vi "compute_statistics_data.vi"() -> ()   [LabVIEW 2020]
uses:
  StatisticsData.ctl
  ComputePhaseSet.lvclass
  WavefrontReconstructionMode.ctl
  HasoData.lvclass
  Phase.lvclass
  Pupil.lvclass
panel:
  out "Wavefront":sgl[][](graph)
  in  "Haso slopes file name":string="Data\\data_phase_computation.has"
  out "error out":errorcluster
  out "Statistics":T1
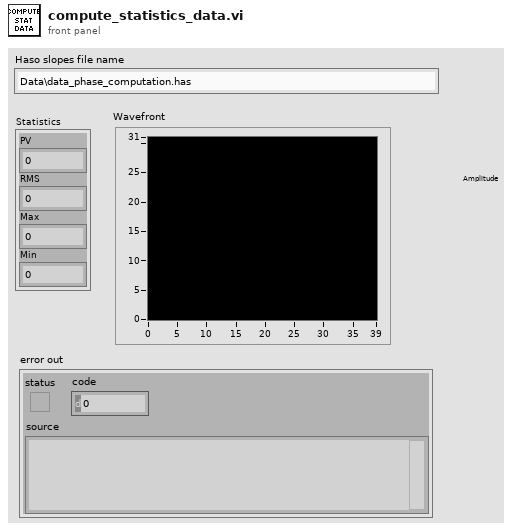
[diagram p1: front panel]
types:
  T1 = typedef "StatisticsData.ctl" = cluster{"PV":sgl, "RMS":dbl, "Max":sgl, "Min":sgl}
  T2 = typedef "WavefrontReconstructionMode.ctl" = enum16{"None", "Modal_Legendre", "Modal_Zernike", "Zonal", "Modal_Zonal_Zernike", "Modal_Zonal_Legendre"}
  T3 = typedef "Point2D.ctl" = cluster{"X":u32, "Y":u32}
  T4 = typedef "Point2Df.ctl" = cluster{"X":sgl, "Y":sgl}
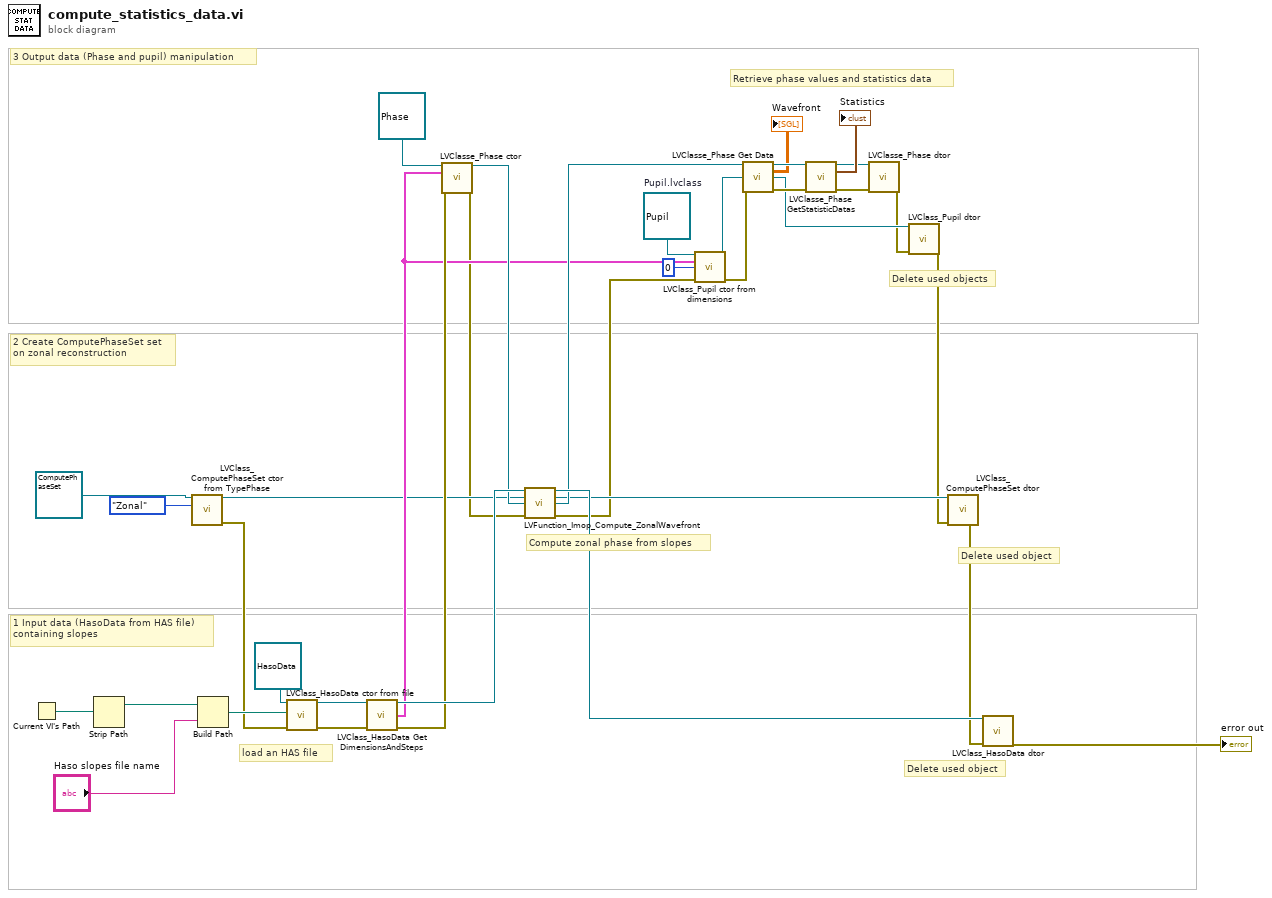
[diagram p0: block diagram]
diagram:
  w16 = refnum<class "Pupil.lvclass"> refnum  # Pupil.lvclass
  # "Compute zonal phase from slopes"
  # "Delete used objects"
  # "Delete used object"
  # "3 Output data (Phase and pupil) manipulation"
  # "2 Create ComputePhaseSet set\non zonal reconstruction"
  # "1 Input data (HasoData from HAS file)\ncontaining slopes"
  # "Delete used object"
  # "Retrieve phase values and statistics data"
  # "load an HAS file"
  n1 = Current VI's Path() -> (path=w24:path)
  n2 = Strip Path(path=w24) -> (stripped path=w21:path)  [unwired: 1 out]
  n3 = call "LVClass_ComputePhaseSet ctor from TypePhase.vi"("ComputePhaseSet in"=refnum<class "ComputePhaseSet.lvclass"> refnum, "TypePhase"=WavefrontReconstructionMode."Zonal") -> ("ComputePhaseSet out"=w10:refnum<class "ComputePhaseSet.lvclass">, "error out"=w20:errorcluster)  [unwired: 12 in]
  n4 = Build Path(base path=w21, name or relative path="Haso slopes file name") -> (appended path=w22:path)
  n5 = call "LVClass_HasoData ctor from file.vi"("HasoData in"=refnum<class "HasoData.lvclass"> refnum, "HAS file path"=w22, "error in (no error)"=w20) -> ("HasoData out"=w33:refnum<class "HasoData.lvclass">, "error out"=w28:errorcluster)  [unwired: 11 in]
  n6 = call "LVClass_HasoData Get DimensionsAndSteps.vi"("HasoData in"=w33, "error in (no error)"=w28) -> ("HasoData out"=w31:refnum<class "HasoData.lvclass">, "Dimensions"=w15:cluster{"size":T3, "steps":T4}, "error out"=w29:errorcluster)  [unwired: 11 in]
  n7 = call "LVClasse_Phase ctor.vi"("Phase in"=refnum<class "Phase.lvclass"> refnum, "Dimensions_um"=w15, "error in (no error)"=w29) -> ("Phase out"=w30:refnum<class "Phase.lvclass">, "error out"=w3:errorcluster)  [unwired: 11 in]
  n8 = call "LVFunction_Imop_Compute_ZonalWavefront.vi"("HasoData.lvclass"=w31, "ComputePhaseSet.lvclass"=w10, "Phase"=w30, "error constant"=w3) -> ("HasoData.lvclass (dup)"=w25:refnum<class "HasoData.lvclass">, "ComputePhaseSet.lvclass 2"=w9:refnum<class "ComputePhaseSet.lvclass">, "Phase"=w19:refnum<class "Phase.lvclass">, "error out"=w2:errorcluster)  [unwired: 8 in]
  n9 = call "LVClass_Pupil ctor from dimensions.vi"("Pupil in"=w16, "Dimensions_um"=w15, "value"=0, "error in (no error)"=w2) -> ("Pupil out"=w13:refnum<class "Pupil.lvclass">, "error out"=w1:errorcluster)  [unwired: 10 in]
  n10 = call "LVClasse_Phase Get Data.vi"("Phase in"=w19, "Pupil"=w13, "error in (no error)"=w1) -> ("Phase out"=w18:refnum<class "Phase.lvclass">, "data"=→"Wavefront":sgl[][], "Pupil (dup)"=w12:refnum<class "Pupil.lvclass">, "error out"=w17:errorcluster)  [unwired: 9 in]
  n11 = call "LVClasse_Phase GetStatisticDatas.vi"("Phase in"=w18, "error in (no error)"=w17) -> ("Phase out"=w26:refnum<class "Phase.lvclass">, "StatisticsData"=→"Statistics":T1, "error out"=w8:errorcluster)  [unwired: 11 in]
  n12 = call "LVClasse_Phase dtor.vi"("Phase in"=w26, "error in (no error)"=w8) -> ("error out"=w4:errorcluster)  [unwired: 12 in, 1 out]
  n13 = call "LVClass_Pupil dtor.vi"("Pupil in"=w12, "error in (no error)"=w4) -> ("error out"=w6:errorcluster)  [unwired: 12 in, 1 out]
  n14 = call "LVClass_ComputePhaseSet dtor.vi"("ComputePhaseSet in"=w9, "error in (no error)"=w6) -> ("error out"=w7:errorcluster)  [unwired: 12 in, 1 out]
  n15 = call "LVClass_HasoData dtor.vi"("HasoData in"=w25, "error in (no error)"=w7) -> ("error out"=→"error out":errorcluster)  [unwired: 12 in, 1 out]
